vi "Pre Launch Init.vi"(11 "Turbo in":refnum<class "Turbo.lvclass">) -> (0 "error out":errorcluster, 3 "Turbo out":refnum<class "Turbo.lvclass">)   [LabVIEW 2015, in "cRIO-Carbondioxide.lvlib" / "CO2-Actor.lvlib" / "Turbo.lvclass"]
doc: "(<B>Filename</B>: Actor Framework.lvlib:Actor.lvclass:Pre Launch Init.vi)\n\nDefines behavior that occurs after the Launch Actor method is invoked but before the actor's Actor Core method begins running.\n\nThe Pre Launch Init method is guaranteed to finish before the Launch Actor method returns to its caller and before the actor itself receives any messages. Any references that the Pre Launch Init method obtains are guaranteed to have the same lifetime as the actor itself. Any errors that the Pre Launch Init method returns will abort the launch.\n\nBy default, this method does nothing. A descendant class may override it to define behavior."
uses:
  Turbo.lvclass
  CO2 Actor Messages/Timeout Msg/Timeout Msg.lvclass
  Turbo.lvclass/Turbo.ctl
  <vilib>/ActorFramework/Actor/Actor.lvclass/Actor.ctl
  <vilib>/ActorFramework/Message Enqueuer/Message Enqueuer.lvclass/Message Enqueuer.ctl
  <vilib>/ActorFramework/Message Enqueuer/Enqueue.vi
  <vilib>/ActorFramework/Actor/Read Self Enqueuer.vi
  <vilib>/ActorFramework/Message Enqueuer/Init from Existing Queue.vi
  <vilib>/ActorFramework/Message Priority Queue/Priority Enqueue.vi
  CO2 Actor/CO2 Actor.lvclass
  CO2 Actor Messages/Launch Nested Actors Msg/Launch Nested Actors Msg.lvclass
  <vilib>/ActorFramework/Message Enqueuer/Message Enqueuer.lvclass
  <vilib>/ActorFramework/Actor/Actor.lvclass
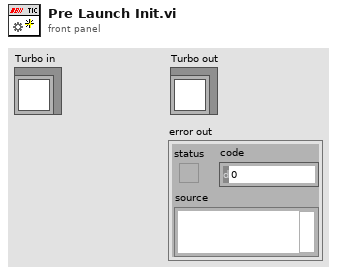
[diagram p1: front panel]
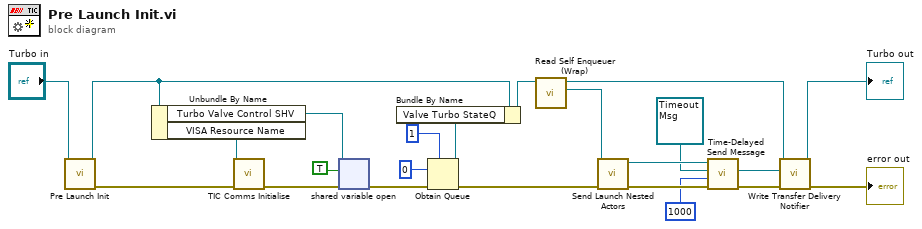
[diagram p0: block diagram]
diagram:
  n1 = call-parent "Pre Launch Init.vi"("CO2 Actor in"="Turbo in") -> ("error out"=w21:errorcluster, "CO2 Actor out"=w22:refnum<class "Turbo.lvclass">)  [unwired: 9 in]
  n2 = Unbundle By Name(w22) -> ("Turbo Valve Control SHV"=w17:refnum<k21>, "VISA Resource Name"=w20:refnum<visa-resource-name>)
  n3 = call <instrlib>:"TIC Comms Initialise.vi"("VISA Resource Name"=w20, "error in (no error)"=w21) -> ("error out"=w18:errorcluster)  [unwired: 12 in, 1 out]
  n4 = shared-variable-open(w17, w18, TRUE) -> (w5:errorcluster)  [unwired: 1 in, 1 out]
  n5 = Obtain Queue(max queue size (-1, unlimited)=1, element data type=u16 0, error in (no error)=w5) -> (queue out=w3:refnum<queue>, error out=w4:errorcluster)  [unwired: 2 in, 1 out]
  n6 = Bundle By Name(cluster=w22, "Valve Turbo StateQ"=w3) -> (w6:refnum<class "Turbo.lvclass">)
  n7 = call "Read Self Enqueuer (Wrap).vi"("CO2 Actor in"=w6) -> ("Actor Framework:Message Enqueuer"=w19:refnum<class "Message Enqueuer.lvclass">, "CO2 Actor out"=w9:refnum<class "Turbo.lvclass">)  [unwired: 9 in]
  n8 = call "Send Launch Nested Actors.vi"("error in (no error)"=w4, "Message Enqueuer"=w19) -> ("error out"=w15:errorcluster, "Message Enqueuer out"=w14:refnum<class "Message Enqueuer.lvclass">)  [unwired: 8 in]
  n9 = call <vilib>:"Time-Delayed Send Message.vi"("error in (no error)"=w15, "Milliseconds To Wait"=1000, "Message"=refnum<class "Timeout Msg.lvclass"> refnum ("Timeout Msg.lvclass"), "Message Enqueuer"=w14) -> ("error out"=w11:errorcluster, "Delivery Notifier"=w7:refnum<notifier>)  [unwired: 6 in]
  n10 = call "Write Transfer Delivery Notifier.vi"("error in (no error)"=w11, "Transfer Delivery Notifier"=w7, "Turbo in"=w9) -> ("error out"=→"error out":errorcluster, "Turbo out"=→"Turbo out":refnum<class "Turbo.lvclass">)  [unwired: 7 in]
